vi "Compute.vi"(8 "error in (no error)":errorcluster, 9 "Data Channels":T2, 10 "x-var":T1, 11 "Aux Data Source in":refnum<class "Aux Data Source.lvclass">) -> (0 "error out":errorcluster, 1 "Add'l Data Channels":T2, 3 "Aux Data Source out":refnum<class "Aux Data Source.lvclass">)   [LabVIEW 2009, in "Aux Data Source.lvclass"]
doc: "Given a data channel and an x-coordinate, compute and return one or more new data channels."
uses:
  Aux Data Source.lvclass
  Instruments/Utility Classes/Readable/Data Channels.ctl
  Instruments/Utility Classes/Readable/Data Channel.ctl
  Instruments/Utility Classes/Readable/Data Point.ctl
  Instruments/Utility Classes/Readable/Readable.lvclass
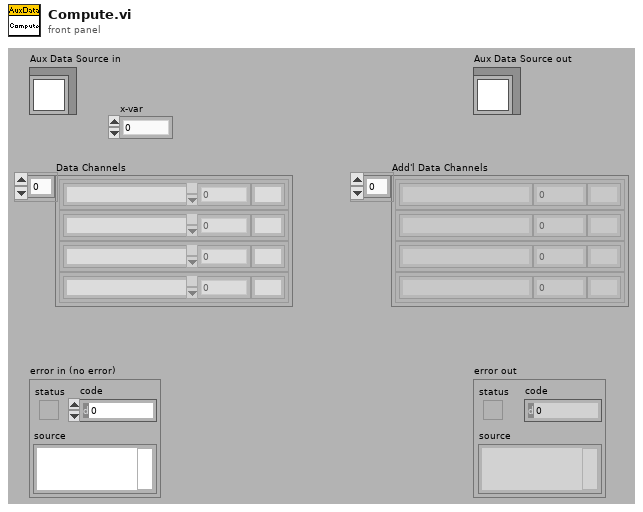
[diagram p1: front panel]
types:
  T1 = typedef "Readable.lvclass/Data Point.ctl" = dbl
  T2 = typedef "Readable.lvclass/Data Channels.ctl" = T3[]
  T3 = typedef "Readable.lvclass/Data Channel.ctl" = cluster{"Name":string, "Data Point":T1, "Unit":string}
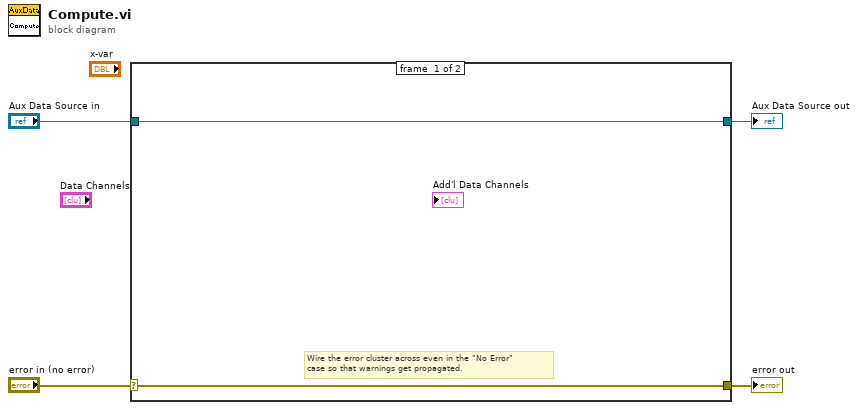
[diagram p0: block diagram]
diagram:
  n1 = case shown="No Error" "error in (no error)" {
    selector: "error in (no error)" -> [w5 w8]
    tunnel: [w5 w8] -> w3
    tunnel: [w6 w7] -> w1
    tunnel: "Aux Data Source in" -> [w6 w7]
    frame #0 {
      # "Wire the error cluster across even in the \"No Error\"\ncase so that warnings get propagated."
    }
    frame #1 {
    }
  }
  "error out" <- w3
  "Aux Data Source out" <- w1
